vi "EditPanel.vi"(8 "error in (no error)":errorcluster, 11 "PLC_Module in":refnum<class "PLC_Module.lvclass">) -> (0 "error out":errorcluster, 3 "PLC_Module out":refnum<class "PLC_Module.lvclass">)   [LabVIEW 2025, in "PLC_Module.lvlib" / "PLC_Module.lvclass"]
uses:
  PLC_Module.lvclass
  PLC_Module.lvclass/PLC_Module.ctl
panel:
  in  "Option":enum16{"Add", "Edit"}(ring)
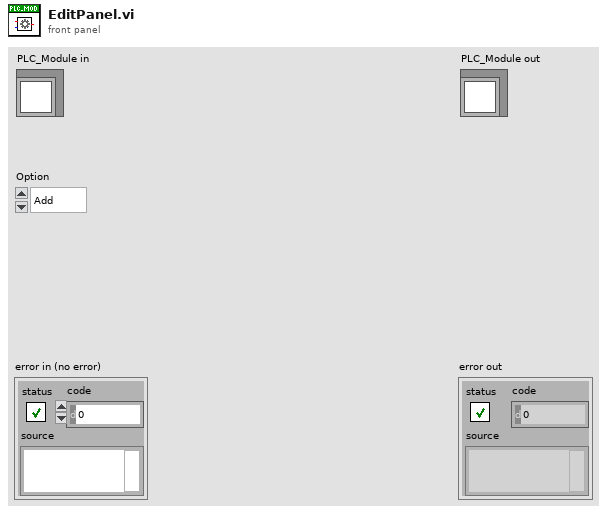
[diagram p1: front panel]
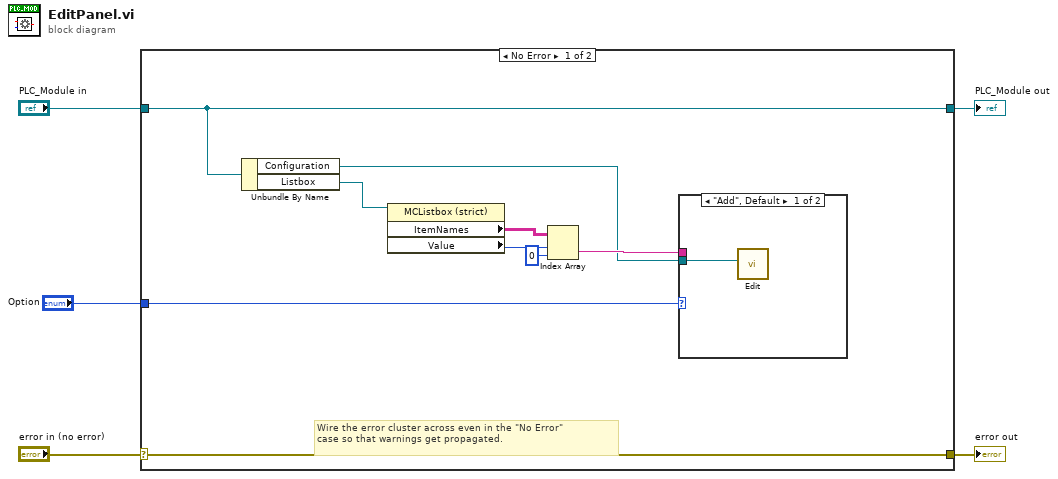
[diagram p0: block diagram]
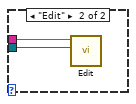
[diagram p2: hidden frame]
diagram:
  n1 = case shown="No Error" "error in (no error)" {
    selector: "error in (no error)" -> [w14 w19]
    tunnel: [w14 w19] -> w4
    tunnel: [w13 w18] -> w2
    tunnel: "PLC_Module in" -> [w13 w18]
    tunnel: "Option" -> [w6 _]
    frame No Error {
      # "Wire the error cluster across even in the \"No Error\"\ncase so that warnings get propagated."
      n2 = Unbundle By Name(w13) -> ("Configuration"=w7:refnum<data-value>, "Listbox"=w12:refnum<vi>)
      n3 = property class="MCListbox (strict)"(reference=w12) -> ("ItemNames"=w11:string[][], "Value"=w10:i32)  [unwired: 1 in, 2 out]
      n4 = Index Array(array=w11, index (row)=w10, index (col)=0 ("disabled index (col)")) -> (element=w8:string)
      n5 = case shown="\"Add\", Default" w6 {
        tunnel: w8 -> [_ w17]
        tunnel: w7 -> [w15 w16]
        frame "Add", Default {
          n6 = call "Edit.vi"("Configuration"=w15) -> ()  [unwired: 11 in]
        }
        frame "Edit" {
          n7 = call "Edit.vi"("Configuration"=w16, "LogicName"=w17) -> ()  [unwired: 10 in]
        }
      }
    }
    frame Error {
    }
  }
  "error out" <- w4
  "PLC_Module out" <- w2
